vi "MongoDB.GetDatabase.vi"(8 "error in (no error)":errorcluster, 10 "databaseName":string, 11 "MongoDB.Connection in":refnum<class "MongoDB.Client.lvclass">) -> (0 "error out":errorcluster, 2 "MongoDB.Database out":refnum<class "MongoDB.Database.lvclass">, 3 "MongoDB.Connection out":refnum<class "MongoDB.Client.lvclass">)   [LabVIEW 2014, in "MongoDB.Client.lvclass"]
uses:
  MongoDB.Client.lvclass
  MongoDB.Database.lvclass
  MongoDB.Client.lvclass/MongoDB.Client.ctl
  C:/Users/Richard/Documents/GitHub/mongo-labview-driver/CSharp/bin/MongoDB.Driver.Legacy.dll
  CSharp/bin/MongoDB.Driver.Legacy.dll
  MongoDB.Database.lvclass/MongoDB.Database.ctl
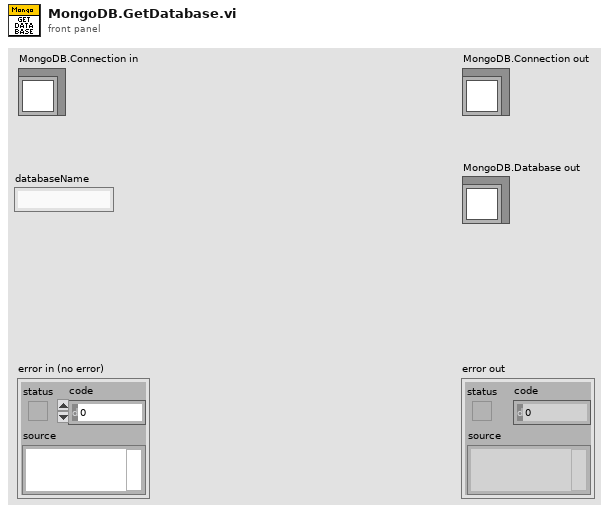
[diagram p1: front panel]
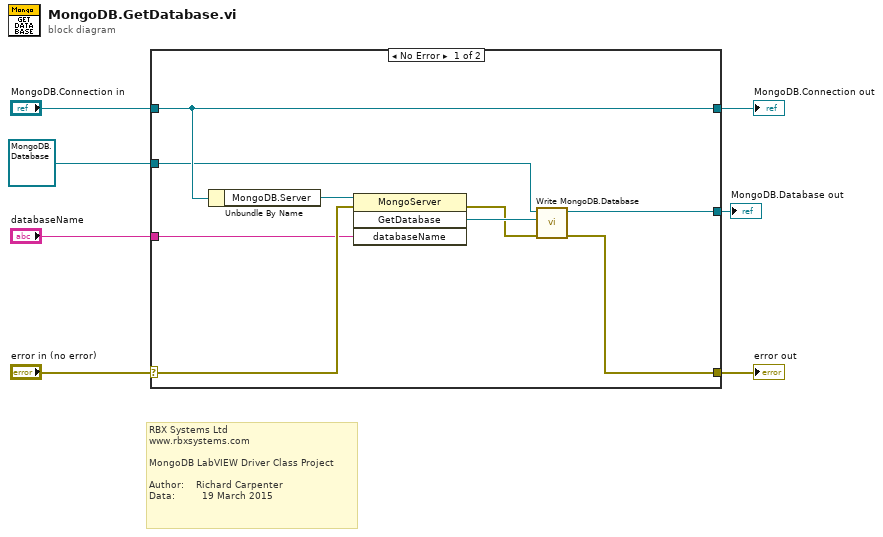
[diagram p0: block diagram]
diagram:
  # "RBX Systems Ltd\nwww.rbxsystems.com\n\nMongoDB LabVIEW Driver Class Project\n\nAuthor:    Richard Carpenter\nData:         19 March 2015"
  n1 = case shown="No Error" "error in (no error)" {
    selector: "error in (no error)" -> [w12 w19]
    tunnel: [w11 w19] -> w4
    tunnel: [w15 w18] -> w6
    tunnel: "MongoDB.Connection in" -> [w15 w18]
    tunnel: [w10 w17] -> w3
    tunnel: "databaseName" -> [w9 _]
    tunnel: refnum<class "MongoDB.Database.lvclass"> refnum ("MongoDB.Database out") -> [w8 w17]
    frame No Error {
      n2 = Unbundle By Name(w15) -> ("MongoDB.Server"=w16:refnum<k24>)
      n3 = invoke class="MongoServer" method="GetDatabase"(reference=w16, error in=w12, "databaseName"=w9) -> (error out=w13:errorcluster, "GetDatabase"=w14:refnum<k24>)  [unwired: 1 in, 2 out]
      n4 = call "Write MongoDB.Database.vi"("error in (no error)"=w13, "MongoDB.Database"=w14, "MongoDB.Database in"=w8) -> ("error out"=w11:errorcluster, "MongoDB.Database out"=w10:refnum<class "MongoDB.Database.lvclass">)  [unwired: 7 in]
    }
    frame Error {
    }
  }
  "error out" <- w4
  "MongoDB.Connection out" <- w6
  "MongoDB.Database out" <- w3
